vi "Host-Fpga-Mac-Top.vi"() -> ()   [LabVIEW 2017]
uses:
  <vilib>/FPGAPlugInAG/PXIe-6592R/niLvFpga_Open_PXIe-6592R.vi
  <vilib>/rvi/interface/common/dynamic/niFpgaDynamicAddResources.vi
  <vilib>/Utility/error.llb/Error Cluster From Error Code.vi
  <vilib>/rvi/errors/niLvFpgaAdjustHostInterfaceError.vi
  <vilib>/FPGAPlugInAG/Dynamic/niLvFpga_Close_Dynamic.vi
  <vilib>/rvi/interface/nirviOpenFPGA/nirviOpenFPGA.xnode
  FPGA Bitfiles/0710GigabitCLIP_FPGATarget_Fpga-Mac-Top_29W8NHw-F2U.lvbitx
  FPGA/MAC/Fpga-Mac-Top.vi
  <vilib>/rvi/interface/nirviReadWriteControl/nirviReadWriteControl.xnode
  <vilib>/rvi/interface/nirviMethod/nirviMethod.xnode
  <vilib>/rvi/interface/nirviCloseFPGA/nirviCloseFPGA.xnode
  NiFpgaLv.dll
  <vilib>/rvi/interface/Simulation/niFpgaSimulationCallBeginRW.vi
  <vilib>/FPGAPlugInAG/Dynamic/niLvFpga_ReadFifo_Dynamic.vi
  <vilib>/rvi/errors/niLvFpgaMergeErrorWithErrorCode.vi
  <vilib>/FPGAPlugInAG/Dynamic/niLvFpga_WriteFifo_Dynamic.vi
panel:
  out "error out 2":errorcluster
  in  "Ethernet II Params":T1={"Destination MAC"=[0, 2, 201, 85, 8, 68], "Source MAC"=[0, 1, 2, 3, 4, 5], "EtherType"=2048} {"Destination MAC" format="%.0x"; "Source MAC" format="%.02x"; "EtherType" format="%.0x"}
  in  "IPv4 Params":T2={"Destination IP"=[10, 0, 1, 100], "Source IP"=[10, 0, 1, 101], "Protocol"=17}
  in  "UDP Params":T3
  in  "Transmit":bool
  out "error out":errorcluster
  in  "Stop":bool
  out "RX Data":i32[](array[numeric])
  in  "MAC local address":u8[](array[numeric])=[0, 1, 2, 3, 4, 5] format="%.0x"
  in  "Promiscuous?":bool=TRUE
  in  "error in":errorcluster
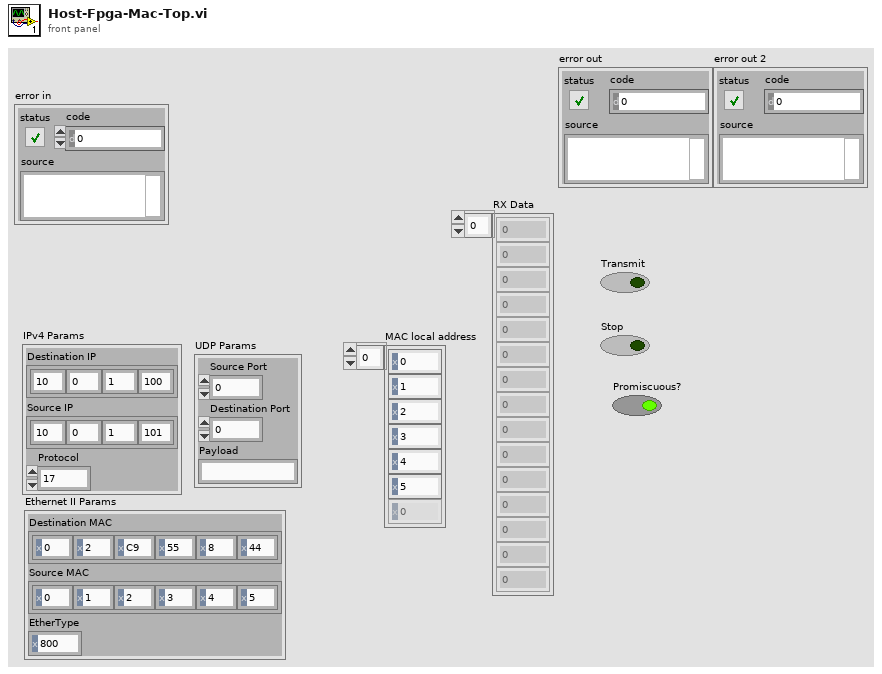
[diagram p1: front panel]
types:
  T1 = cluster{"Destination MAC":u8[], "Source MAC":u8[], "EtherType":u16}
  T2 = cluster{"Destination IP":u8[], "Source IP":u8[], "Protocol":u8}
  T3 = cluster{"Source Port":u16, "Destination Port":u16, "Payload":string}
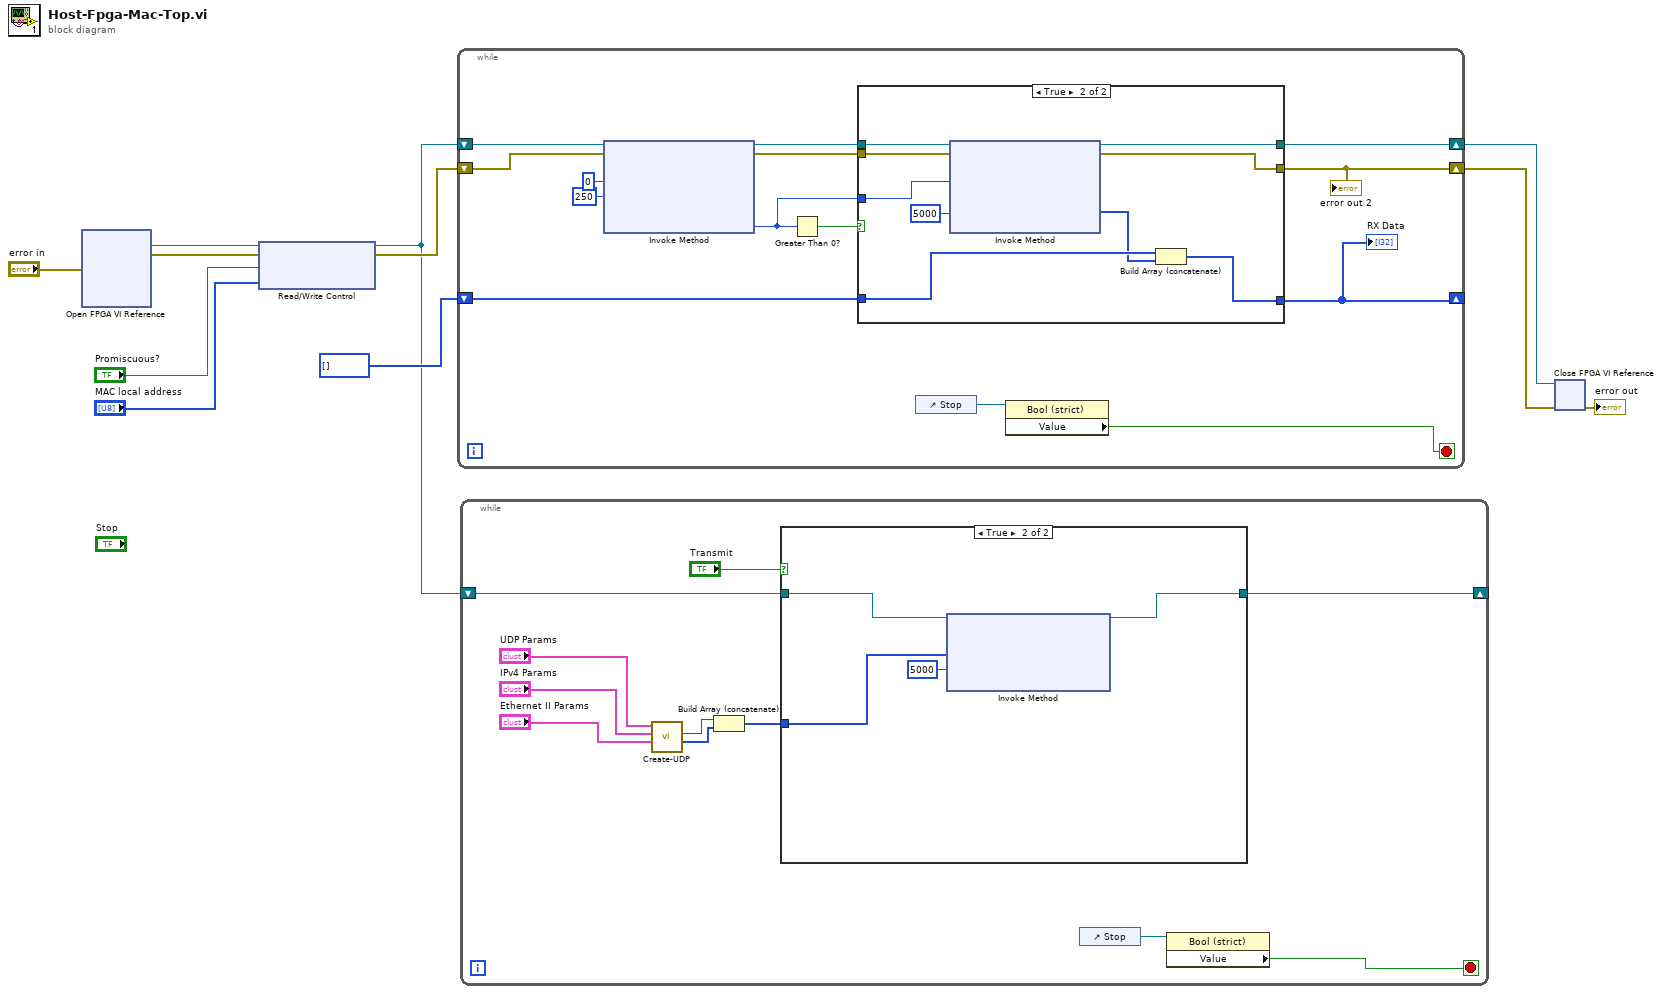
[diagram p0: block diagram]
diagram:
  n1 = xnode "Open FPGA VI Reference"("error in"="error in") -> ("FPGA VI Reference Out"=w10:refnum<k20>, "error out"=w9:errorcluster)  [unwired: 1 in]
  n2 = xnode "Read/Write Control"("FPGA VI Reference In"=w10, "error in"=w9, "Promiscuous?"="Promiscuous?", "MAC local address"="MAC local address") -> ("FPGA VI Reference Out"=w1:refnum<k20>, "error out"=w6:errorcluster)
  n3 = while {
    shift-right: [w16] -> w3
    shift-left: w6 -> [w24]
    shift-right: [w17] -> w4
    shift-left: w1 -> [w25]
    shift-right: [w14] -> _
    shift-left: i32[] [] -> [w15]
    stop <- w13 stop-if-true
    n4 = xnode "Invoke Method"("FPGA VI Reference In"=w25, "error in"=w24, "Number of Elements"=u32 0, "Timeout (ms)"=250) -> ("FPGA VI Reference Out"=w18:refnum<k20>, "error out"=w19:errorcluster, "Elements Remaining"=w20:u32)  [unwired: 1 out]
    n5 = Greater Than 0?(x=w20) -> (x > 0?=w21:bool)
    n6 = case shown="True" w21 {
      tunnel: w20 -> [_ w37]
      tunnel: w19 -> [w27 w36]
      tunnel: w18 -> [w28 w35]
      tunnel: [w28 w33] -> w17
      tunnel: [w27 w32] -> w16
      tunnel: [w26 w29] -> w14
      tunnel: w15 -> [w26 w31]
      frame False {
      }
      frame True {
        n7 = xnode "Invoke Method"("FPGA VI Reference In"=w35, "error in"=w36, "Number of Elements"=w37, "Timeout (ms)"=5000) -> ("FPGA VI Reference Out"=w33:refnum<k20>, "error out"=w32:errorcluster, "Data"=w30:u8[])  [unwired: 1 out]
        n8 = Build Array (concatenate)(w31, w30) -> (w29:i32[])
      }
    }
    "RX Data" <- w14
    "error out 2" <- w16
    n9 = control-ref of="Stop"() -> (w12:refnum<vi>)
    n10 = property class="Bool (strict)"(reference=w12) -> ("Value"=w13:bool)  [unwired: 1 in, 2 out]
  }
  n11 = while {
    shift-right: [w41] -> _
    shift-left: w1 -> [w42]
    stop <- w44 stop-if-true
    n12 = call "Create-UDP.vi"("Ethernet II Params"="Ethernet II Params", "IPv4 Params"="IPv4 Params", "UDP Params"="UDP Params") -> ("Ethernet Frame\nU64"=w39:u64[], "Ethernet Frame\nsize"=w40:i32)  [unwired: 6 in, 1 out]
    n13 = Build Array (concatenate)(w40, w39) -> (w38:u64[])
    n14 = case shown="True" "Transmit" {
      tunnel: w42 -> [w49 w53]
      tunnel: [w49 w50] -> w41
      tunnel: w38 -> [_ w52]
      frame False {
      }
      frame True {
        n15 = xnode "Invoke Method"("FPGA VI Reference In"=w53, "Data"=w52, "Timeout (ms)"=5000) -> ("FPGA VI Reference Out"=w50:refnum<k20>)  [unwired: 1 in, 2 out]
      }
    }
    n16 = control-ref of="Stop"() -> (w45:refnum<vi>)
    n17 = property class="Bool (strict)"(reference=w45) -> ("Value"=w44:bool)  [unwired: 1 in, 2 out]
  }
  n18 = xnode "Close FPGA VI Reference"("FPGA VI Reference In"=w4, "error in"=w3) -> ("error out"=→"error out":errorcluster)
